vi "overlay arc.vi"(8 "error in (no error)":errorcluster, 10 "Search Arcs":T2[](array[typedef]) {"Edge Info"."Distance (Real-World)" format="%.2f"; "Edge Info"."Location (Real-World)"."Y" format="%.2g"; "Edge Info"."Location (Real-World)"."X" format="%.2f"; "Edge Info"."Noise" format="%.2f"; "Edge Info"."Location (Pixel)"."Y" format="%.2g"; "Edge Info"."Location (Pixel)"."X" format="%.2f"; "Edge Info"."Strength" format="%.2f"; "Edge Info"."Distance (Pixel)" format="%.2f"}, 11 "Image in":T1) -> (0 "error out":errorcluster, 3 "Image out":T1)   [LabVIEW 2019]
uses:
  <vilib>/vision/Measure.llb/Search Arc.ctl
  <vilib>/vision/Measure.llb/Edge New.ctl
  <vilib>/vision/Image Controls.llb/IMAQ Image.ctl
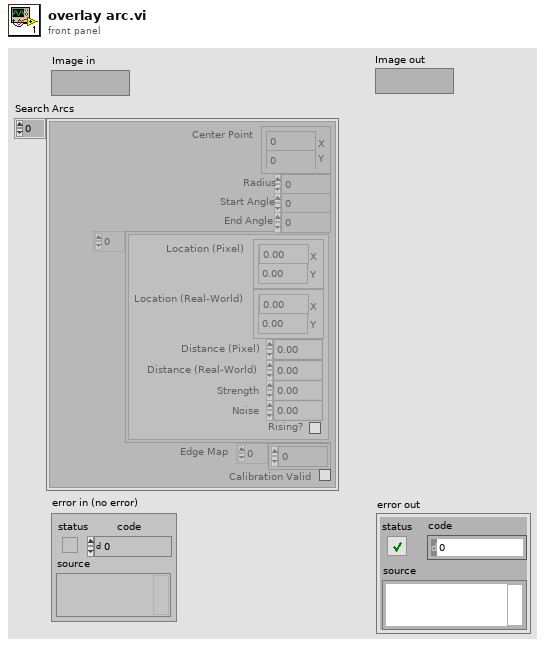
[diagram p1: front panel]
types:
  T1 = typedef "IMAQ Image.ctl" = refnum<image>
  T2 = typedef "Search Arc.ctl" = cluster{"Center Point":cluster{"X":sgl, "Y":sgl}, "Radius":dbl, "Start Angle":dbl, "End Angle":dbl, "Edge Info":T3[], "Edge Map":dbl[], "Calibration Valid":bool}
  T3 = typedef "Edge New.ctl" = cluster{"Location (Pixel)":cluster{"X":sgl, "Y":sgl}, "Location (Real-World)":cluster{"X":sgl, "Y":sgl}, "Distance (Pixel)":dbl, "Distance (Real-World)":dbl, "Strength":dbl, "Noise":dbl, "Rising?":bool}
  T4 = cluster{"Left":i32, "Top":i32, "Right":i32, "Bottom":i32}
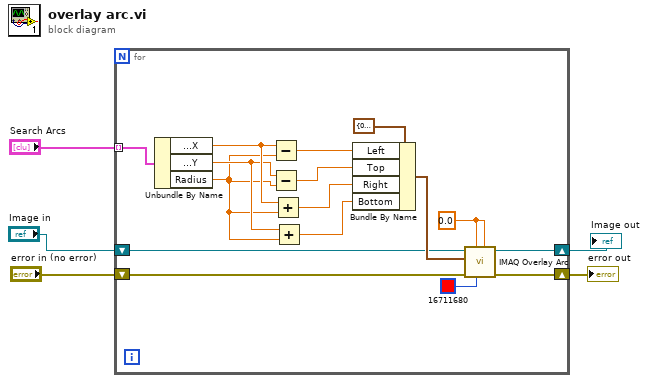
[diagram p0: block diagram]
diagram:
  n1 = for {
    tunnel: "Search Arcs" -> [w21] mode=indexing
    shift-right: [w9] -> w2
    shift-left: "error in (no error)" -> [w10]
    shift-right: [w6] -> w1
    shift-left: "Image in" -> [w11]
    w7 = 0.0 ("Start Angle (degrees)")
    n2 = Unbundle By Name(w21) -> ("Center Point.X"=w19:sgl, "Center Point.Y"=w18:sgl, "Radius"=w17:dbl)
    n3 = Subtract(x=w19, y=w17) -> (x-y=w16:dbl)
    n4 = Subtract(x=w18, y=w17) -> (x-y=w15:dbl)
    n5 = Add(x=w19, y=w17) -> (x+y=w14:dbl)
    n6 = Add(x=w18, y=w17) -> (x+y=w13:dbl)
    n7 = Bundle By Name(cluster=T4 {"Left"=0, "Top"=0, "Right"=0, "Bottom"=0} ("Bounding Rectangle"), "Left"=w16, "Top"=w15, "Right"=w14, "Bottom"=w13) -> (w12:T4)
    n8 = call "IMAQ Overlay Arc"("End Angle (degrees)"=w7, "Color"=u32 16711680, "Start Angle (degrees)"=w7, "error in (no error)"=w10, "Bounding Rectangle"=w12, "Image"=w11) -> ("error out"=w9:errorcluster, "Image Out"=w6:T1)  [unwired: 4 in]
  }
  "error out" <- w2
  "Image out" <- w1
